vi "array2ROI.vi"(10 "length":i32[](array[numeric]), 11 "array":dbl[][][](array[numeric])) -> (2 "ROI":T1(array[cluster]), 3 "corner":dbl[][][](array[numeric]))   [LabVIEW 2017]
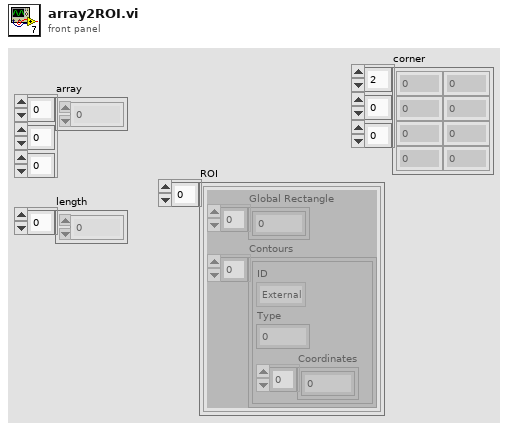
[diagram p1: front panel]
types:
  T1 = cluster{"Global Rectangle":dbl[], "Contours":cluster{"ID":enum32{"External", "Internal"}, "Type":u32, "Coordinates":i32[]}[]}[]
  T2 = typedef "ROI Descriptor" = cluster{"Global Rectangle":i32[], "Contours":cluster{"ID":enum32{"External", "Internal"}, "Type":u32, "Coordinates":i32[]}[]}
  T3 = cluster{"ID":enum32{"External", "Internal"}, "Type":u32, "Coordinates":i32[]}
  T4 = cluster{"ID":enum32{"External", "Internal"}, "Type":u32, "Coordinates":i32[]}[]
  T5 = cluster{dbl[], cluster{"ID":enum32{"External", "Internal"}, "Type":u32, "Coordinates":i32[]}[]}
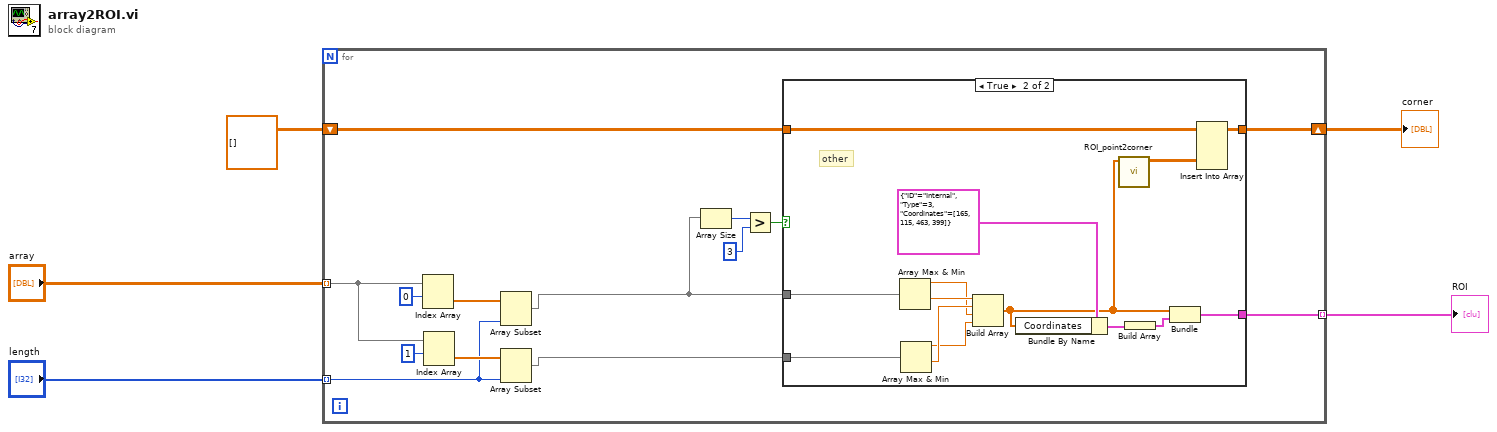
[diagram p0: block diagram]
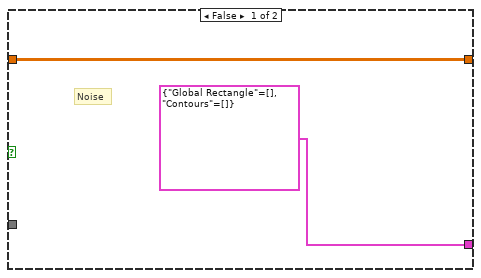
[diagram p2: hidden frame]
diagram:
  n1 = for {
    tunnel: [w19] -> w3 mode=indexing
    shift-right: [w14] -> w1
    shift-left: dbl[][][] [] ("Array 2") -> [w15]
    tunnel: "array" -> [w13] mode=indexing
    tunnel: "length" -> [w8] mode=indexing
    n2 = Index Array "Index Array"(array=w13, index (row)=0) -> (element=w10:dbl[])  [unwired: 1 in]
    n3 = Index Array(array=w13, index (row)=1) -> (element=w9:dbl[])  [unwired: 1 in]
    n4 = Array Subset "Array Subset"(array=w10, length=w8) -> (w7:dbl[])  [unwired: 1 in]
    n5 = Array Subset(array=w9, length=w8) -> (w6:dbl[])  [unwired: 1 in]
    n6 = Array Size(array=w7) -> (size(s)=w17:i32)
    n7 = Greater?(x=w17, y=3) -> (0:w18:bool)
    n8 = case shown="True" w18 {
      tunnel: w7 -> [_ w35]
      tunnel: [T2 {"Global Rectangle"=[], "Contours"=[]} ("ROI Descriptor") w27] -> w19
      tunnel: w15 -> [w20 w26]
      tunnel: [w20 w25] -> w14
      tunnel: w6 -> [_ w24]
      frame False {
        # "Noise"
      }
      frame True {
        # "other"
        n9 = Array Max & Min(array=w35) -> (max value=w32:dbl, min value=w34:dbl)  [unwired: 2 out]
        n10 = Array Max & Min(array=w24) -> (max value=w31:dbl, min value=w33:dbl)  [unwired: 2 out]
        n11 = Build Array(w34, w33, w32, w31) -> (w23:dbl[])
        n12 = Bundle By Name(cluster=T3 {"ID"=enum."Internal", "Type"=3, "Coordinates"=[165, 115, 463, 399]}, "Coordinates"=w23) -> (w30:T3)
        n13 = call "ROI_point2corner.vi"("appended array"=w23) -> ("Array"=w22:dbl[][])  [unwired: 10 in]
        n14 = Build Array(w30) -> (w28:T4)
        n15 = Bundle(w23, w28) -> (w27:T5)  [unwired: 1 in]
        n16 = Insert Into Array(array=w26, new element=w22) -> (w25:dbl[][][])  [unwired: 3 in]
      }
    }
  }
  "ROI" <- w3
  "corner" <- w1
